vi "GenCalibrationRefsMultiMix.vi"(7 "Misselaneous Parems":T2, 8 "Base Dilution":dbl, 9 "Mix Sequence Array":bool[][](array[boolean]), 10 "Valves":u16[](array[ring]) items=["A1", "A2", "A3", "A4", "B1", "B2", "B3", "B4", "B5", "B6", "B7", "B8", "A5"], 11 "Pressure Group":enum16{"1", "2", "3", "4"}[](array[ring])=[enum."3", enum."3", enum."3", enum."3", enum."4", enum."4", enum."4", enum."4", enum."1", enum."1", enum."1", enum."1", enum."1"]) -> (1 "Possible Water Mix Ratios":dbl[](array[numeric]), 2 "Calibration Refs":T1)   [LabVIEW 2016]
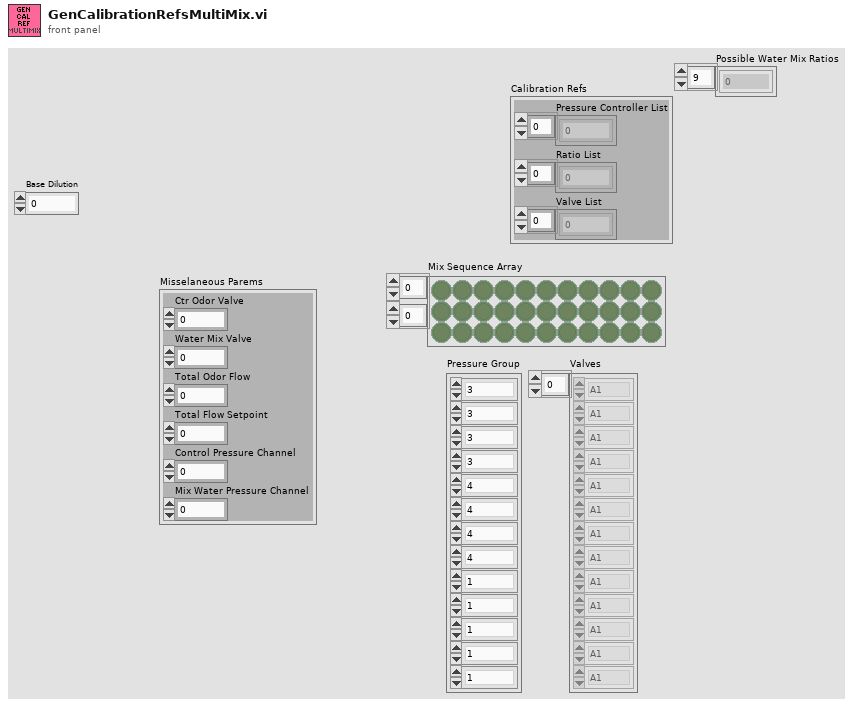
[diagram p1: front panel]
types:
  T1 = cluster{"Pressure Controller List":u8[], "Ratio List":dbl[], "Valve List":u16[]}
  T2 = cluster{"Ctr Odor Valve":u16, "Water Mix Valve":u16, "Total Odor Flow":dbl, "Total Flow Setpoint":dbl, "Control Pressure Channel":u16, "Mix Water Pressure Channel":u16}
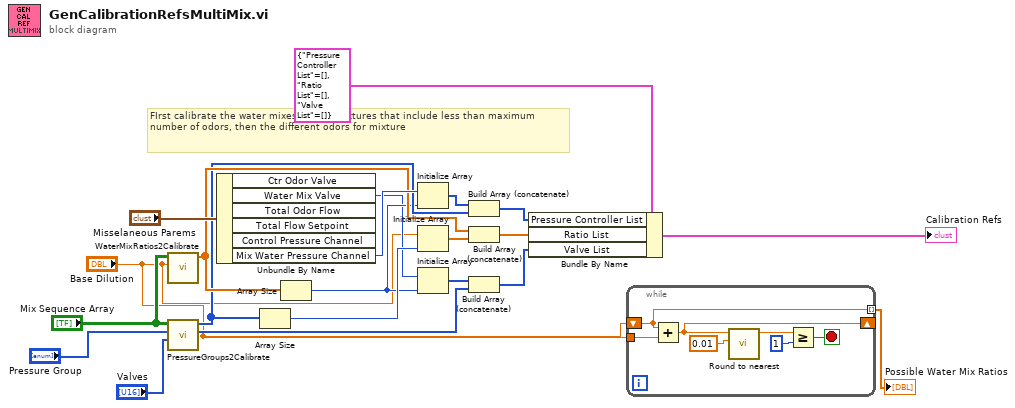
[diagram p0: block diagram]
diagram:
  # "FIrst calibrate the water mixes for the mixtures that include less than maximum number of odors, then the different odors for mixture"
  n1 = call "WaterMixRatios2Calibrate.vi"("Base Dilution"="Base Dilution", "Mix Sequence Array"="Mix Sequence Array") -> ("waterRatio"=w14:dbl[])  [unwired: 8 in, 1 out]
  n2 = call "PressureGroups2Calibrate.vi"("Valves"="Valves", "Pressure Group"="Pressure Group", "Mix Sequence Array"="Mix Sequence Array") -> ("Valves 2 Calibrate"=w8:u16[], "Pressure Groups to Calibrate"=w13:u16[])  [unwired: 7 in]
  n3 = Unbundle By Name("Misselaneous Parems") -> ("Water Mix Valve"=w5:u16, "Mix Water Pressure Channel"=w16:u16)  [unwired: 4 out]
  n4 = Array Size(array=w13) -> (size(s)=w12:i32)
  n5 = Array Size(array=w14) -> (size(s)=w6:i32)
  n6 = Initialize Array(w16, w6) -> (w15:u16[])
  n7 = Initialize Array("Base Dilution", w12) -> (w11:dbl[])
  n8 = Initialize Array(w5, w6) -> (w4:u16[])
  n9 = Build Array (concatenate)(w15, w13) -> (w9:u16[])
  n10 = Build Array (concatenate)(w14, w11) -> (w10:dbl[])
  n11 = Build Array (concatenate)(w4, w8) -> (w7:u16[])
  n12 = Bundle By Name(cluster=T1 {"Pressure Controller List"=[], "Ratio List"=[], "Valve List"=[]} ("Calibration Refs"), "Pressure Controller List"=w9, "Ratio List"=w10, "Valve List"=w7) -> (→"Calibration Refs":T1)
  n13 = while {
    tunnel: "Base Dilution" -> [w28]
    shift-right: [w23] -> _
    shift-left: "Base Dilution" -> [w27]
    tunnel: [w27] -> w2 mode=indexing
    stop <- w25 stop-if-true
    n14 = Add(x=w27, y=w28) -> (x+y=w23:dbl)
    n15 = call "Round to nearest.vi"("Round to nearest"=0.01, "Number"=w23) -> ("Rounded"=w22:dbl)  [unwired: 9 in]
    n16 = Greater Or Equal?(x=w22, y=u16 1) -> (x >= y?=w25:bool)
  }
  "Possible Water Mix Ratios" <- w2
